vi "CRYCal Perceptual Rub&buzz TSR.vi"(6 "Fs":dbl=44100.0, 8 "TSR params":T1={"FSamp"=44100.0, "FStart"=20.0, "FStop"=20000.0, "NOffset"=0.0, "MStop"=132741.0, "MStart"=441.0, "NHarm"=19152.386651933408, "Tsamp"=2.2675736961451248e-05, "Amplit"=0.5, "Sweep Time"=1.0} {"Sweep Time" format="%.2f"; "Amplit" format="%.2f"; "FStop" format="%.2f"; "FStart" format="%.2f"; "FSamp" format="%.2f"; "Tsamp" format="%.2f"; "NHarm" format="%.2f"; "MStart" format="%.2f"; "MStop" format="%.2f"; "NOffset" format="%.2f"}, 10 "Response":dbl[](array[numeric]) format="%.2f", 11 "Stimulus":dbl[](array[numeric]) format="%.2f") -> (2 "EHS + NL":dbl[](array[numeric]), 3 "Frequency":dbl[](array[numeric]))   [LabVIEW 2013]
panel:
  out "EHS + NL PHON":cluster{"Fc":dbl[], dbl[]}(graph)
  out "NL Loudness 2":cluster{"Fc":dbl[], "y out":dbl[]}[](graph)
  out "Response EWeight dBSPL":cluster{"Freq":dbl[], "EpR":dbl[]}[](graph)
  out "Stimulus EWeight dBSPL":cluster{"Freq":dbl[], "EpR":dbl[]}[](graph)
  out "NL Loudness":cluster{"Fc":dbl[], dbl[]}(graph)
  out "Adapt":cluster{"Freq":dbl[], "EpR":dbl[]}[](graph)
  out "Response dBSPL":cluster{"Fc":dbl[], dbl[]}(graph)
  out "Stimulus dBSPL":cluster{"Fc":dbl[], dbl[]}(graph)
  out "EHS Phon":cluster{"Fc":dbl[], dbl[]}(graph)
  out "EHS + NL SPL":cluster{"Fc":dbl[], dbl[]}(graph)
  out "EHS":cluster{"Fc":dbl[], dbl[]}(graph)
  out "Response Wave":waveform(dbl)(graph)
  out "Stimulus Wave":waveform(dbl)(graph)
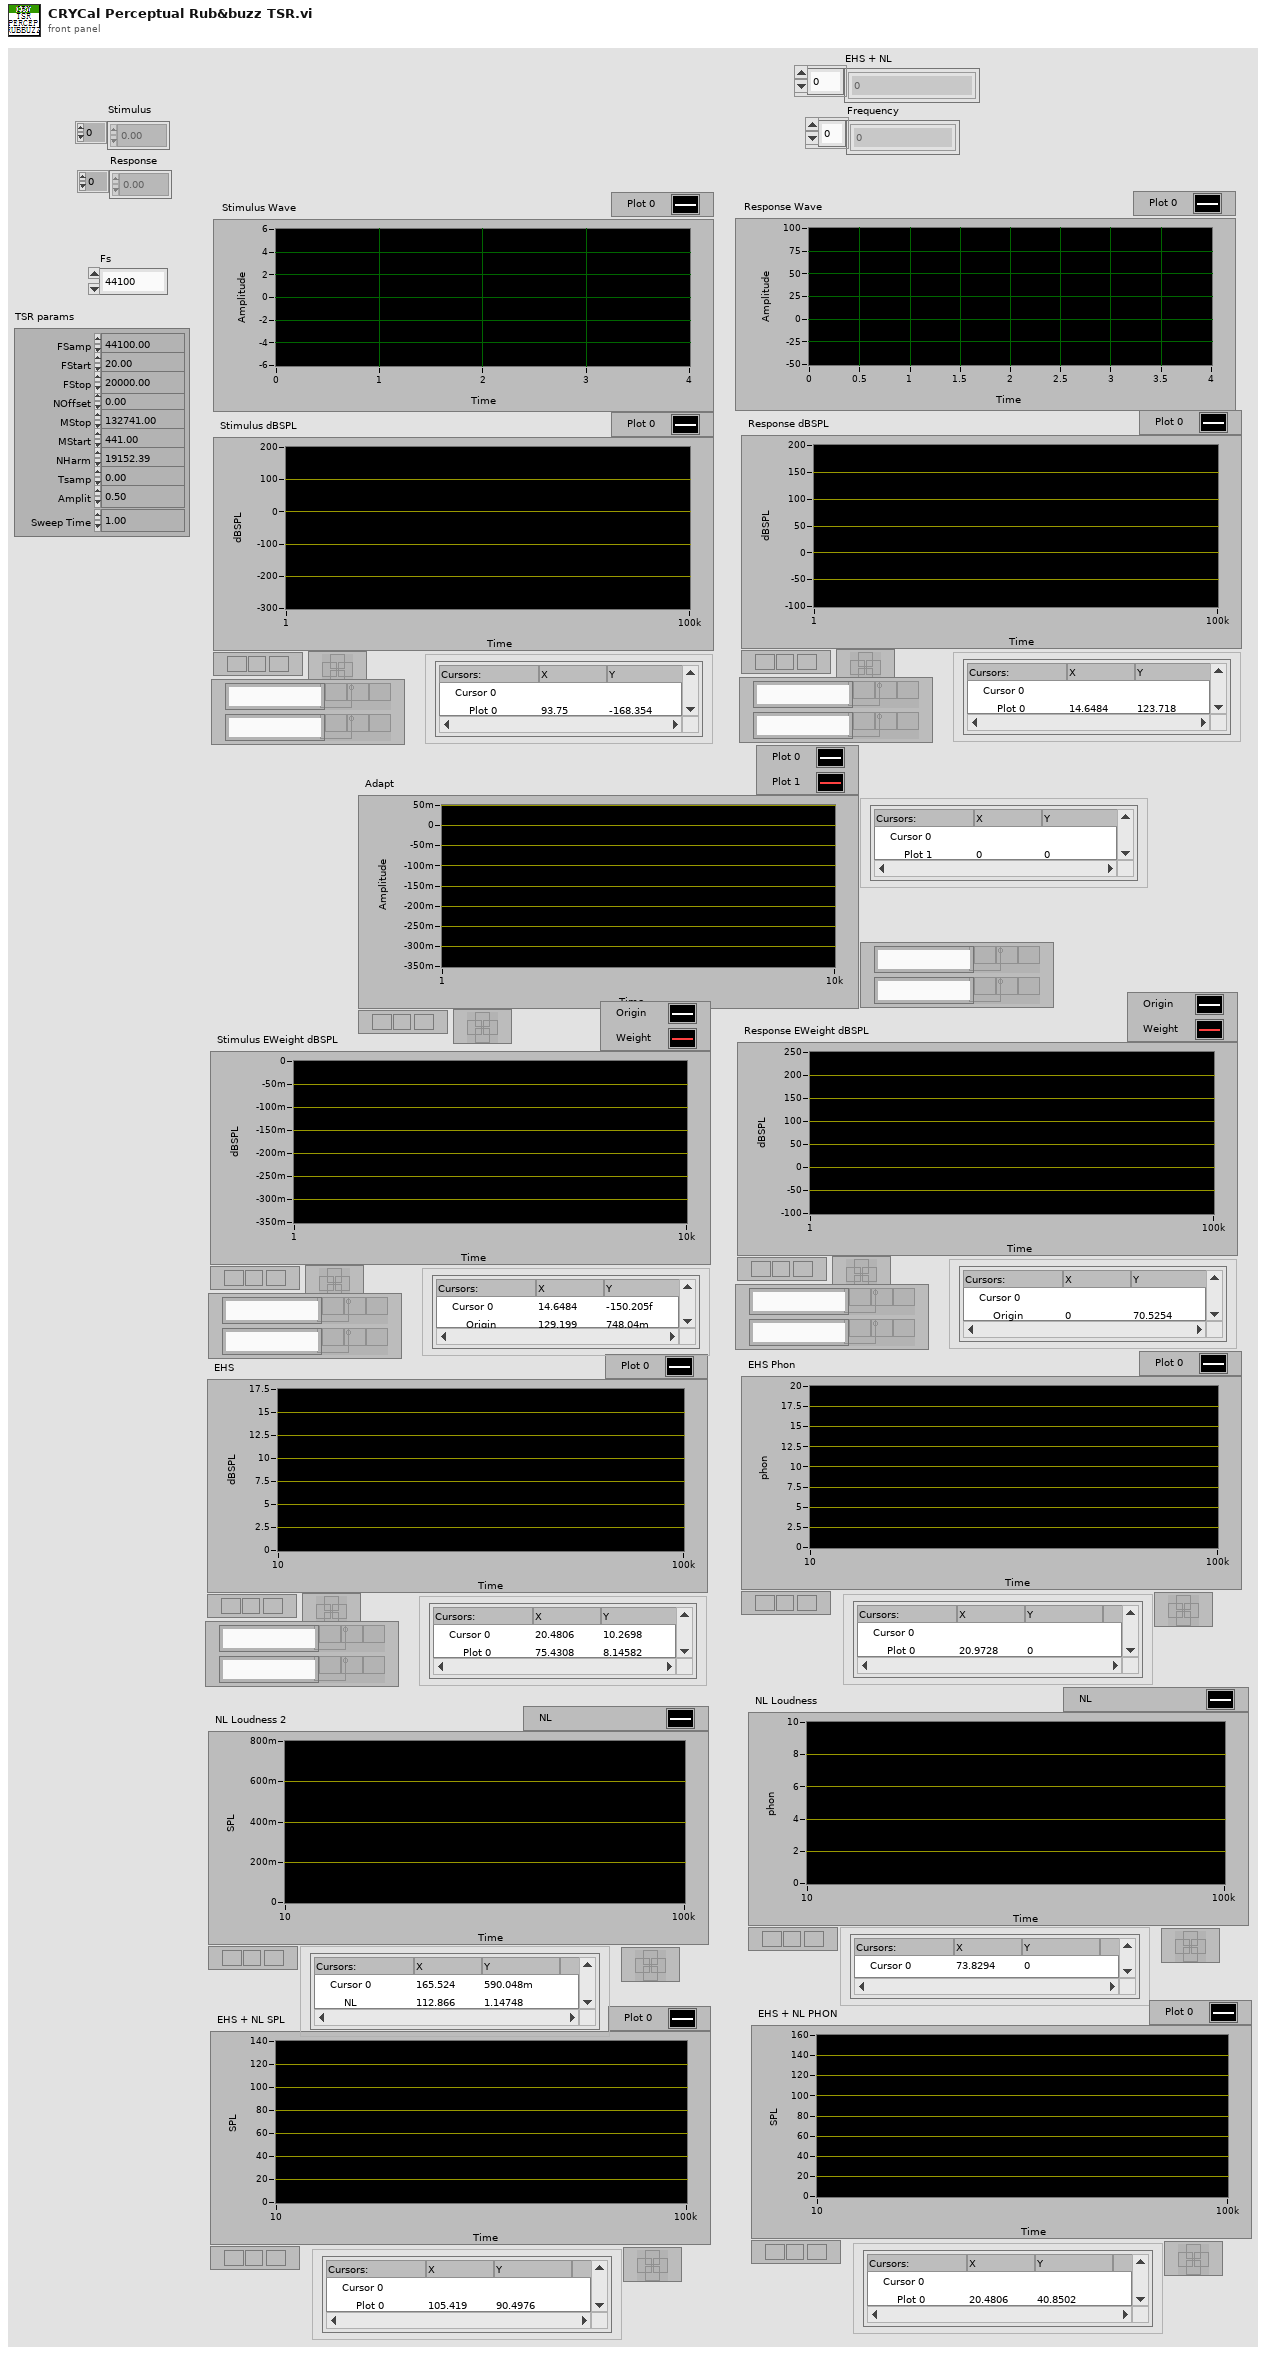
[diagram p1: front panel]
types:
  T1 = cluster{"FSamp":dbl, "FStart":dbl, "FStop":dbl, "NOffset":dbl, "MStop":dbl, "MStart":dbl, "NHarm":dbl, "Tsamp":dbl, "Amplit":dbl, "Sweep Time":dbl}
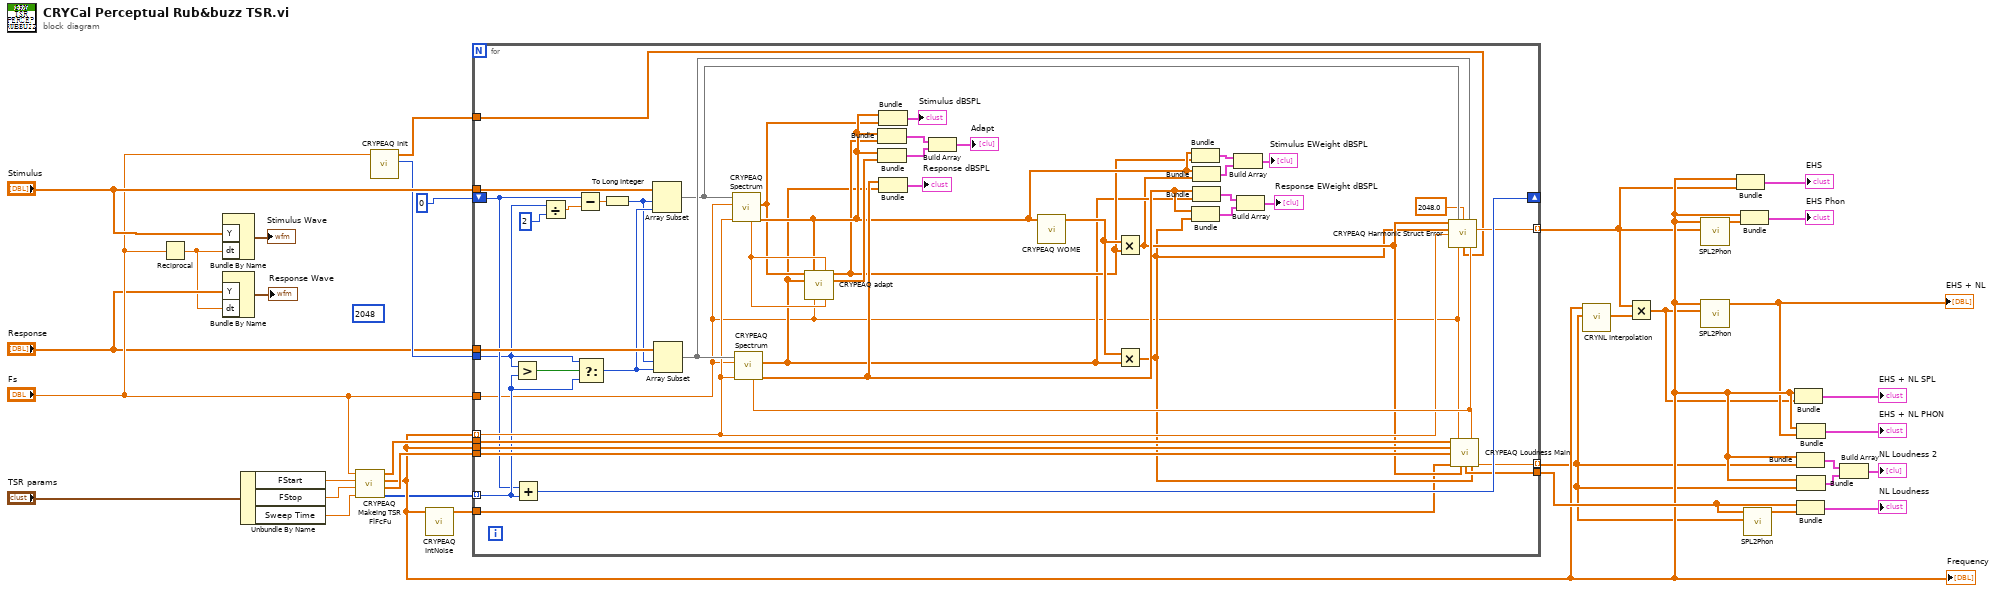
[diagram p0: block diagram]
diagram:
  (unwired) 2048
  n1 = Reciprocal(x="Fs") -> (1/x=w5:dbl)
  n2 = Bundle By Name("Y"="Stimulus", "dt"=w5) -> (→"Stimulus Wave":waveform(dbl))  [unwired: 1 in]
  n3 = Bundle By Name("Y"="Response", "dt"=w5) -> (→"Response Wave":waveform(dbl))  [unwired: 1 in]
  n4 = Unbundle By Name("TSR params") -> ("FStart"=w30:dbl, "FStop"=w28:dbl, "Sweep Time"=w34:dbl)
  n5 = call "CRYPEAQ Makeing TSR FlFcFu.vi"("Sweep time"=w34, "Fstop"=w28, "Fstart"=w30, "Fs"="Fs") -> ("Fu Index"=w19:i32[], "Fu"=w29:dbl[], "Fc"=w21:dbl[], "Fl"=w31:dbl[])  [unwired: 3 in]
  "Frequency" <- w21
  n6 = call "CRYPEAQ Init.vi"("Fs"="Fs") -> ("Block Size"=w22:i32, "Hanning Window"=w23:dbl[])  [unwired: 9 in]
  n7 = call "CRYPEAQ IntNoise.vi"("fc"=w21) -> ("EIN"=w25:dbl[])  [unwired: 10 in]
  n8 = for {
    tunnel: "Stimulus" -> [w76]
    tunnel: "Response" -> [w75]
    tunnel: "Fs" -> [w46]
    shift-right: [w81] -> _
    shift-left: 0 -> [w56]
    tunnel: w19 -> [w58] mode=indexing
    tunnel: w21 -> [w67] mode=indexing
    tunnel: w31 -> [w80]
    tunnel: w29 -> [w79]
    tunnel: w21 -> [w71]
    tunnel: [w78] -> w17 mode=indexing
    tunnel: [w54] -> w2 mode=indexing
    tunnel: [w64] -> w27
    tunnel: w25 -> [w53]
    tunnel: w23 -> [w49]
    tunnel: w22 -> [w47]
    n9 = Greater?(x=w47, y=w58) -> (0:w77:bool)
    n10 = Add(x=w56, y=w58) -> (x+y=w81:i32)
    n11 = Divide(x=w47, y=2) -> (x/y=w51:dbl)
    n12 = Subtract(x=w56, y=w51) -> (x-y=w55:dbl)
    n13 = Select(t=w47, s=w77, f=w58) -> (s? t:f=w57:i32)
    n14 = To Long Integer(number=w55) -> (32bit integer=w50:i32)
    n15 = Array Subset(array=w76, index=w50, length=w57) -> (w65:dbl[])
    n16 = Array Subset(array=w75, index=w50, length=w57) -> (w70:dbl[])
    n17 = call "CRYPEAQ Spectrum.vi"("Freq"=w67, "Fs"=w46, "X"=w65) -> ("Freq"=w66:dbl[], "dBSPL Spectrum"=w63:dbl[], "FFT Size"=w74:dbl)  [unwired: 5 in, 1 out]
    n18 = call "CRYPEAQ Spectrum.vi"("Freq"=w67, "Fs"=w46, "X"=w70) -> ("Freq"=w73:dbl[], "dBSPL Spectrum"=w61:dbl[], "FFT Size"=w72:dbl)  [unwired: 5 in, 1 out]
    n19 = call "CRYPEAQ adapt.vi"("EhsR"=w63, "fc"=w66, "Nc"=w74, "EhsT"=w61, "Fs"=w46, "NF"=w74) -> ("EpR"=w62:dbl[], "EpT"=w68:dbl[])  [unwired: 8 in]
    n20 = Bundle("Freq"=w66, "EpR"=w62) -> (w37:cluster{"Freq":dbl[], "EpR":dbl[]})  [unwired: 1 in]
    n21 = Bundle("Freq"=w66, "EpT"=w68) -> (w36:cluster{"Freq":dbl[], "EpT":dbl[]})  [unwired: 1 in]
    n22 = Bundle("Freq"=w66, "dBSPL Spectrum"=w63) -> (→"Stimulus dBSPL":cluster{"Freq":dbl[], "dBSPL Spectrum":dbl[]})  [unwired: 1 in]
    n23 = Bundle("Freq"=w73, "dBSPL Spectrum"=w61) -> (→"Response dBSPL":cluster{"Freq":dbl[], "dBSPL Spectrum":dbl[]})  [unwired: 1 in]
    n24 = Build Array(w37, w36) -> (→"Adapt":cluster{"Freq":dbl[], "EpT":dbl[]}[])
    n25 = call "CRYPEAQ WOME.vi"("f"=w66) -> ("W2"=w69:dbl[])  [unwired: 10 in]
    n26 = Multiply(x=w69, y=w62) -> (x*y=w60:dbl[])
    n27 = Multiply(x=w69, y=w61) -> (x*y=w59:dbl[])
    n28 = Bundle("Freq"=w66, "EpR"=w62) -> (w42:cluster{"Freq":dbl[], "EpR":dbl[]})  [unwired: 1 in]
    n29 = Bundle("Freq"=w73, w59) -> (w45:cluster{"Freq":dbl[], dbl[]})  [unwired: 1 in]
    n30 = Bundle("Freq"=w66, w60) -> (w41:cluster{"Freq":dbl[], dbl[]})  [unwired: 1 in]
    n31 = Bundle("Freq"=w73, "dBSPL Spectrum"=w61) -> (w44:cluster{"Freq":dbl[], "dBSPL Spectrum":dbl[]})  [unwired: 1 in]
    n32 = Build Array(w42, w41) -> (→"Stimulus EWeight dBSPL":cluster{"Freq":dbl[], "EpR":dbl[]}[])
    n33 = Build Array(w44, w45) -> (→"Response EWeight dBSPL":cluster{"Freq":dbl[], "dBSPL Spectrum":dbl[]}[])
    n34 = call "CRYPEAQ Harmonic Struct Error.vi"("Level Adaptation -> EarWeighted Stimulus"=w60, "Stimulus"=w65, "Correlation Point Number"=2048.0, "Response"=w70, "EarWeighted Response"=w59, "Fc Hz"=w67, "Fs"=w46, "Hanning Window"=w49, "NF"=w72) -> ("EHS"=w78:dbl)  [unwired: 6 in]
    n35 = call "CRYPEAQ Loudness Main.vi"("Fl"=w80, "Fs"=w46, "NF"=w72, "Fc"=w71, "Fu"=w79, "Internal Noise"=w53, "X2R"=w60, "X2T"=w59) -> ("fc"=w64:dbl[], "NL"=w54:dbl)  [unwired: 4 in, 2 out]
  }
  n36 = call "CRYNL Interpolation.vi"("y in"=w2, "x in"=w21) -> ("y out"=w1:dbl[])  [unwired: 9 in]
  n37 = Multiply(x=w17, y=w1) -> (x*y=w16:dbl[])
  n38 = call "SPL2Phon.vi"("SPL in"=w17, "Frequency in"=w21) -> ("Phon out"=w13:dbl[])  [unwired: 9 in]
  n39 = call "SPL2Phon.vi"("SPL in"=w16, "Frequency in"=w21) -> ("Phon out"=w20:dbl[])  [unwired: 9 in]
  "EHS + NL" <- w20
  n40 = Bundle("Fc"=w21, w17) -> (→"EHS":cluster{"Fc":dbl[], dbl[]})  [unwired: 1 in]
  n41 = Bundle("Fc"=w21, "Phon out"=w13) -> (→"EHS Phon":cluster{"Fc":dbl[], "Phon out":dbl[]})  [unwired: 1 in]
  n42 = call "SPL2Phon.vi"("SPL in"=w2, "Frequency in"=w27) -> ("Phon out"=w9:dbl[])  [unwired: 9 in]
  n43 = Bundle("Fc"=w21, w16) -> (→"EHS + NL SPL":cluster{"Fc":dbl[], dbl[]})  [unwired: 1 in]
  n44 = Bundle("Fc"=w21, w2) -> (w8:cluster{"Fc":dbl[], dbl[]})  [unwired: 1 in]
  n45 = Bundle("fc"=w27, "Phon out"=w9) -> (→"NL Loudness":cluster{"fc":dbl[], "Phon out":dbl[]})  [unwired: 1 in]
  n46 = Bundle("Fc"=w21, "Phon out"=w20) -> (→"EHS + NL PHON":cluster{"Fc":dbl[], "Phon out":dbl[]})  [unwired: 1 in]
  n47 = Bundle("Fc"=w21, w2) -> (w7:cluster{"Fc":dbl[], dbl[]})  [unwired: 1 in]
  n48 = Build Array(w8, w7) -> (→"NL Loudness 2":cluster{"Fc":dbl[], dbl[]}[])
